vi "End Game.vi"(11 "Square in":refnum<class "Square.lvclass">) -> ()   [LabVIEW 2020, in "SquareBattle.lvlib" / "Square.lvclass"]
uses:
  Square.lvclass
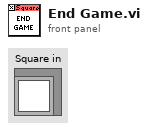
[diagram p1: front panel]
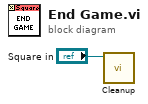
[diagram p0: block diagram]
diagram:
  n1 = call-dynamic "Cleanup.vi"("Square"="Square in") -> ()  [unwired: 11 in]
